vi "Simple Client.vi"() -> ()   [LabVIEW 2020]
uses:
  source/Client/Client/Client.lvclass
  source/Client/Client/Get - DBL.vi
  source/Client/Client/Put - DBL.vi
panel:
  out "doubled value":dbl
  out "value":dbl
  in  "PV name":string="DEV:FLOAT64"
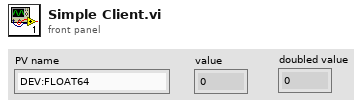
[diagram p1: front panel]
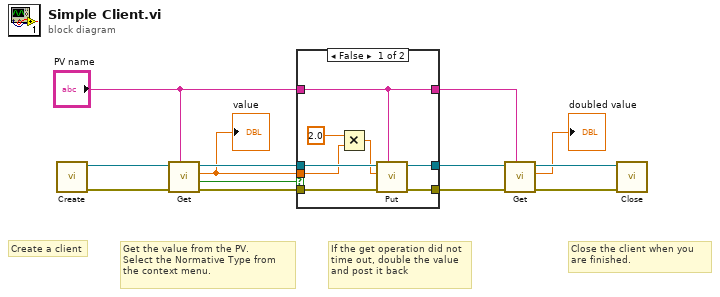
[diagram p0: block diagram]
diagram:
  # "Close the client when you are finished."
  # "If the get operation did not time out, double the value and post it back"
  # "Get the value from the PV.\nSelect the Normative Type from the context menu."
  # "Create a client"
  n1 = call "Create.vi"() -> ("error out"=w11:errorcluster, "Client out"=w12:refnum<class "Client.lvclass">)  [unwired: 10 in]
  n2 = call-poly "Get.vi"("PV name"="PV name", "error in (no error)"=w11, "Client in"=w12) -> ("error out"=w9:errorcluster, "timed out?"=w8:bool, "value"=w7:dbl, "Client out"=w10:refnum<class "Client.lvclass">)  [unwired: 4 in, 1 out]
  "value" <- w7
  n3 = case shown="False" w8 {
    tunnel: w7 -> [w16 _]
    tunnel: [w21 w24] -> w5
    tunnel: [w20 w23] -> w6
    tunnel: w10 -> [w19 w24]
    tunnel: w9 -> [w18 w23]
    tunnel: "PV name" -> [w17 w22]
    tunnel: [w17 w22] -> w2
    frame False {
      n4 = Multiply(x=2.0, y=w16) -> (x*y=w14:dbl)
      n5 = call-poly "Put.vi"("PV name"=w17, "error in (no error)"=w18, "value in"=w14, "Client in"=w19) -> ("error out"=w20:errorcluster, "Client out"=w21:refnum<class "Client.lvclass">)  [unwired: 5 in, 1 out]
    }
    frame True {
    }
  }
  n6 = call-poly "Get.vi"("PV name"=w2, "error in (no error)"=w6, "Client in"=w5) -> ("error out"=w3:errorcluster, "value"=→"doubled value":dbl, "Client out"=w4:refnum<class "Client.lvclass">)  [unwired: 4 in, 2 out]
  n7 = call "Close.vi"("error in (no error)"=w3, "Client in"=w4) -> ()  [unwired: 9 in, 1 out]
